vi "Find Test Cases in LVProj.vi"(8 "error in (no error)":errorcluster, 11 "Project Path":path) -> (0 "error out":errorcluster, 2 "Test Class paths":path[](array[path]))   [LabVIEW 2020, in "Test Suite Factory.lvclass"]
uses:
  LUnit Test Case/LUnit Test Case.lvclass
  Test Suite Factory.lvclass
  Test Suite Factory.lvclass/Test Suite Factory.ctl
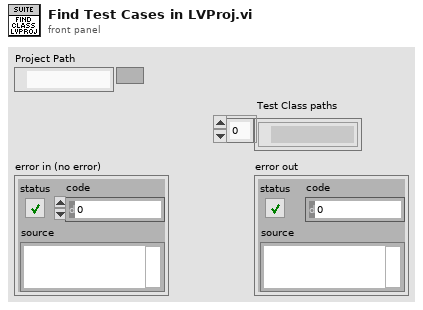
[diagram p1: front panel]
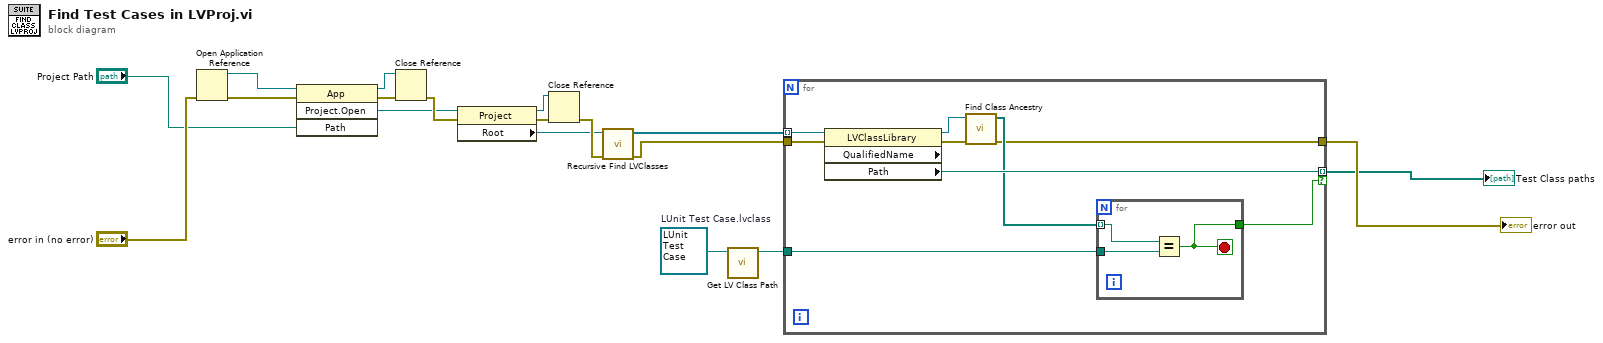
[diagram p0: block diagram]
diagram:
  w2 = refnum<class "LUnit Test Case.lvclass"> refnum  # LUnit Test Case.lvclass
  n1 = Open Application Reference(8:"error in (no error)") -> (0:w8:errorcluster, 3:w7:refnum<vi>)  [unwired: 3 in]
  n2 = invoke class="App" method="Project.Open"(reference=w7, error in=w8, "Path"="Project Path") -> (reference out=w10:refnum<vi>, error out=w9:errorcluster, "Project:Open"=w11:refnum<vi>)  [unwired: 1 in, 1 out]
  n3 = Close Reference(reference=w10, error in (no error)=w9) -> (error out=w12:errorcluster)
  n4 = property class="Project"(reference=w11, error in=w12) -> (reference out=w18:refnum<vi>, error out=w13:errorcluster, "Root"=w3:refnum<vi>)
  n5 = Close Reference(reference=w18, error in (no error)=w13) -> (error out=w17:errorcluster)
  n6 = call "Recursive Find LVClasses.vi"("error in (no error)"=w17, "reference"=w3) -> ("error out"=w4:errorcluster, "Class References"=w14:refnum<vi>[])  [unwired: 8 in]
  n7 = call <vilib>:"Get LV Class Path.vi"("object"=w2) -> ("class path"=w1:path)  [unwired: 9 in, 1 out]
  n8 = for {
    tunnel: w14 -> [w27] mode=indexing
    tunnel: w4 -> [w26]
    tunnel: [w20] -> w16
    tunnel: [w25] -> w5 mode=indexing if=w23
    tunnel: w1 -> [w24]
    n9 = property class="LVClassLibrary" props=["QualifiedName", "Path"](reference=w27, error in=w26) -> (reference out=w19:refnum<vi>, error out=w21:errorcluster, "Path"=w25:path)  [unwired: 1 out]
    n10 = call "Find Class Ancestry.vi"("error in (no error)"=w21, "reference in"=w19) -> ("error out"=w20:errorcluster, "Class Ancestry"=w22:path[])  [unwired: 8 in]
    n11 = for {
      tunnel: w22 -> [w29] mode=indexing
      tunnel: w24 -> [w30]
      tunnel: [w28] -> w23
      stop <- w28 stop-if-true
      n12 = Equal?(x=w29, y=w30) -> (x = y?=w28:bool)
    }
  }
  "error out" <- w16
  "Test Class paths" <- w5
